vi "Action Worker Mode Example.vi"() -> ()   [LabVIEW 2017]
uses:
  user.lib/_NEVSTOP/Communicable State Machine(CSM)/_Support/Typedef/_CSM_Response Source Message.ctl
  user.lib/_NEVSTOP/Communicable State Machine(CSM)/_Support/Typedef/_CSM_MODE.ctl
  user.lib/_NEVSTOP/Communicable State Machine(CSM)/AdvanceAPI/CSM - Break Down Multiple States String.vi
  user.lib/_NEVSTOP/Communicable State Machine(CSM)/AdvanceAPI/CSM - Compact Multiple States.vi
  user.lib/_NEVSTOP/Communicable State Machine(CSM)/AdvanceAPI/CSM - Make String Arguments Safe.vi
  user.lib/_NEVSTOP/Communicable State Machine(CSM)/AdvanceAPI/CSM - Keywords.vi
  user.lib/_NEVSTOP/Communicable State Machine(CSM)/_Support/CSMQ/_CSMOFGV.vi
  user.lib/_NEVSTOP/Communicable State Machine(CSM)/_Support/FGV-BroadcastRegistry/global-CSMQ FGV Change Flag.vi
  user.lib/_NEVSTOP/Communicable State Machine(CSM)/Communicable State Machine.lvlib
panel:
  in  "All?":bool
  out "Array":T2(array[cluster])
  out ">> Response Source Message >>":T3
  in  "DoSth: Error -> Worker":bool
  in  "DoSth: Error -@ Worker":bool
  in  "Macro: Exit -> Worker":bool
  in  "Macro: Exit -@ Worker":bool
  in  "DoSth: DoA -@ Worker":bool
  out "State History":string
  in  "DoSth: DoA -> Worker":bool
  # "Overview:\n\nThis demonstrates the worker mode in the CSM framework. Worker mode involves starting multiple clonable instances of CSM, which work together as sub-modules. Normally, if we use the same name for cloneable modules, a critical error will occur in the subsequently started instance. To distinguish it from normal cases, CSM uses a # postfix in module names. Suppose the workers are named with \"worker#\". If you try to send a message to \"worker\", the first idle instance will respond to the message. The term \"FIRST IDLE\" refers to using a fairy queue for waiting instances. From outside, you won't even know that 4 worker instances are running. All concepts of CSM remain unchanged in worker mode, including sync/async/status messages.\n\nIn this example, 4 worker instances of “worker” are running in the background. Please refer to the history log to identify which instance processed your message."
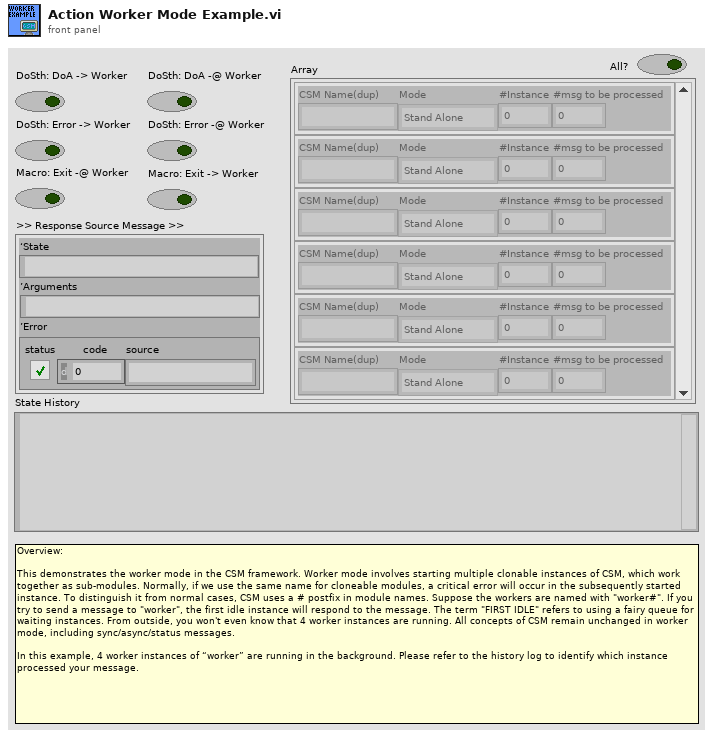
[diagram p1: front panel]
types:
  T1 = typedef "Communicable State Machine.lvlib/_CSM_MODE.ctl" = enum16{"Not Exist", "Stand Alone", "CSM", "Worker Agent", "Worker", "Chain", "Chain Node"}
  T2 = cluster{"CSM Name(dup)":string, "Mode":T1, "#Instance":i32, "#msg to be processed":i32}[]
  T3 = typedef "Communicable State Machine.lvlib/_CSM_Response Source Message.ctl" = cluster{"‘State":string, "’Arguments":string, "’Error":errorcluster}
  T4 = enum32{"Invalid", "Standard", "Closed", "Hidden", "Minimized", "Maximized"}
  T5 = enum32{"invalid app kind", "Development System", "Run Time System", "Student Edition", "Embedded LabVIEW", "Evaluation", "Custom"}
  T6 = cluster{"Current VI Reference":refnum<vi>, "Close Panel on Exit?":bool}
  T7 = cluster{"Core":cluster{"Current VI Reference":refnum<vi>, "Close Panel on Exit?":bool}, "Your Boolean data":bool, "Your string data":string}
  T8 = cluster{"CSM Name(dup)":string, "Mode":T1, "#Instance":i32, "#msg to be processed":i32}
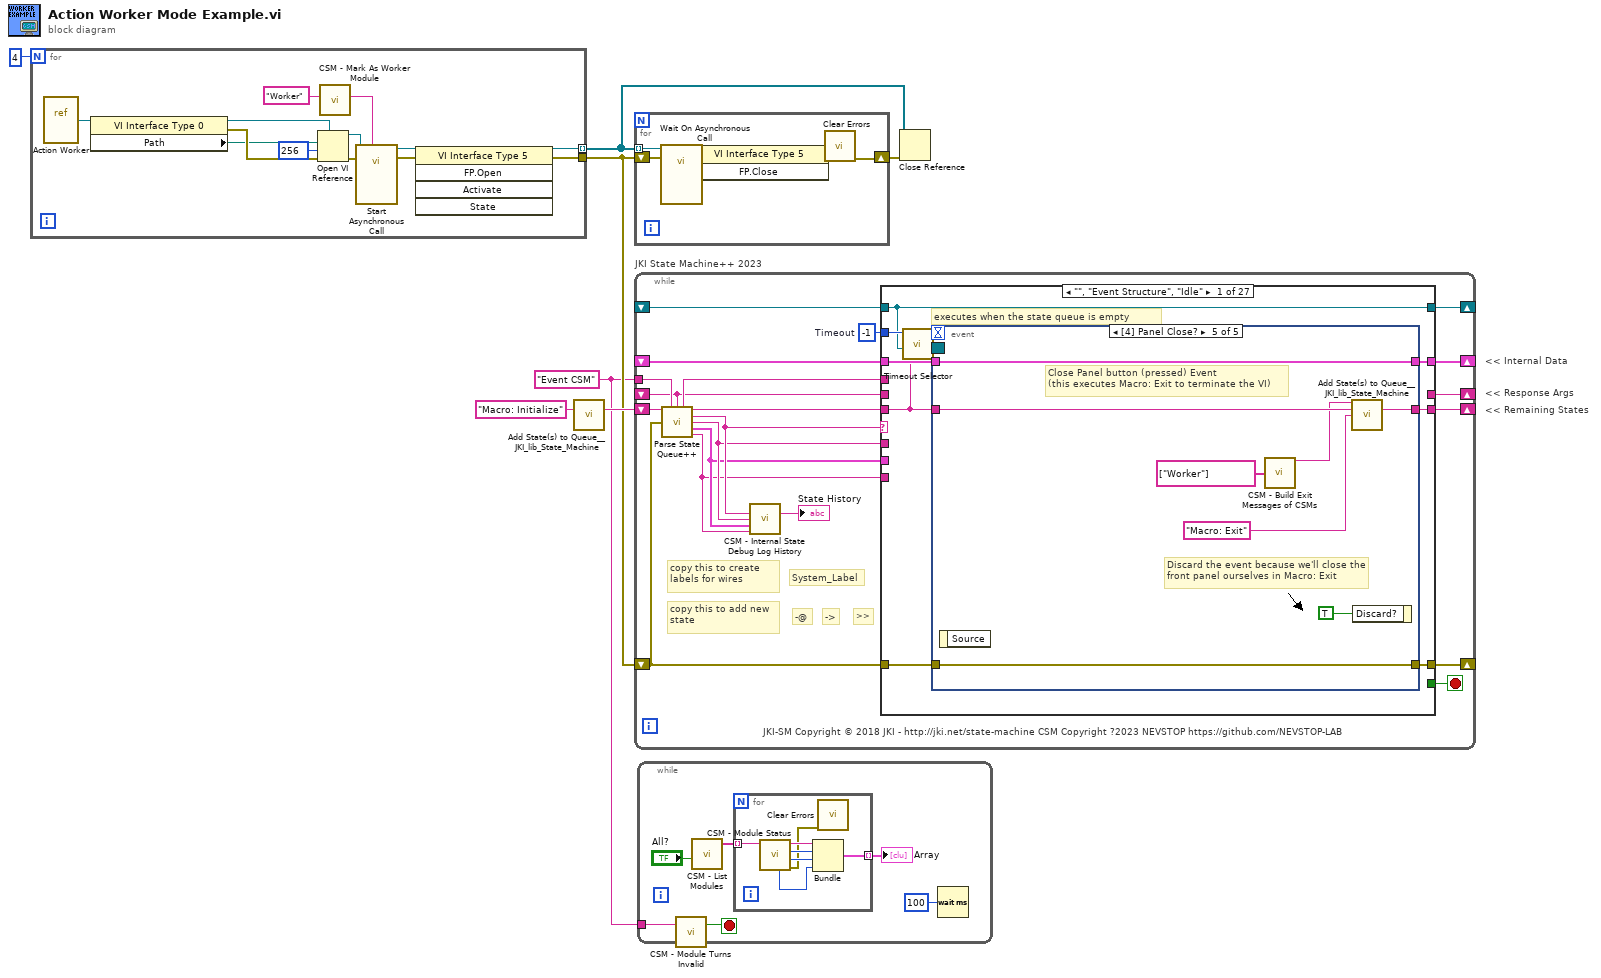
[diagram p0: block diagram]
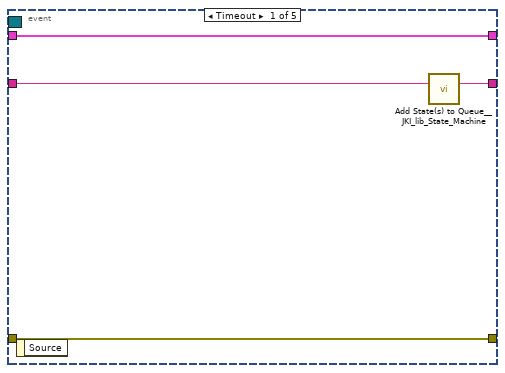
[diagram p2: hidden frame]
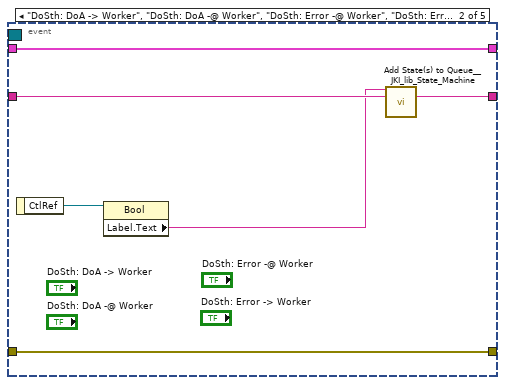
[diagram p3: hidden frame]
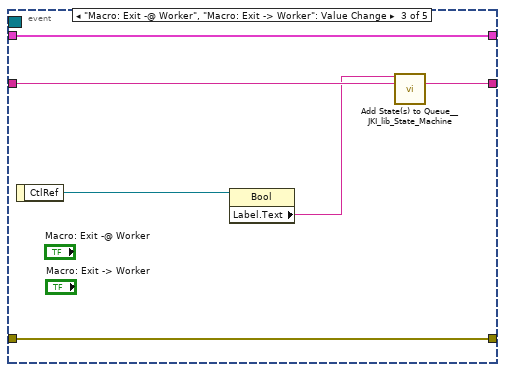
[diagram p4: hidden frame]
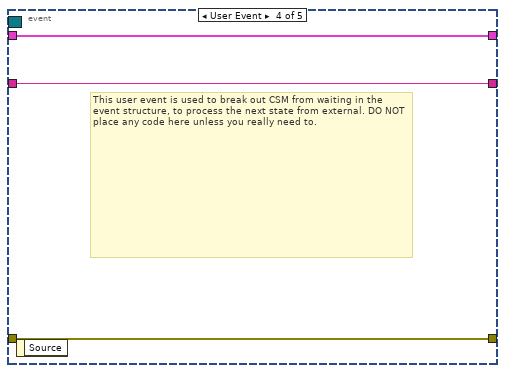
[diagram p5: hidden frame]
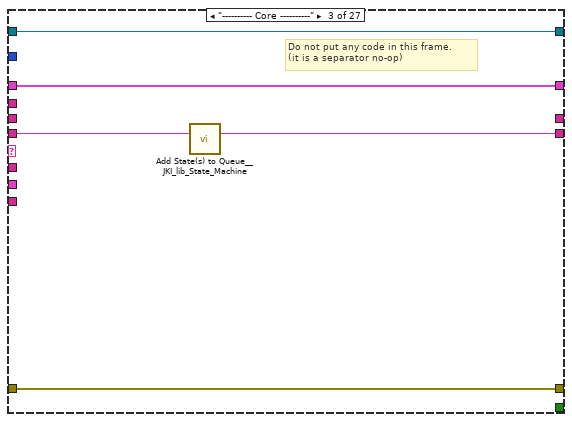
[diagram p7: hidden frame]
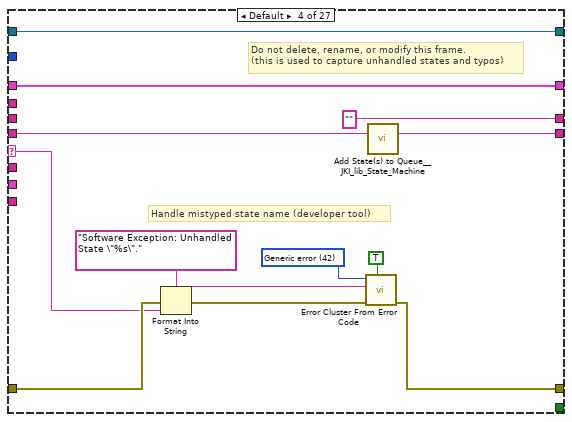
[diagram p8: hidden frame]
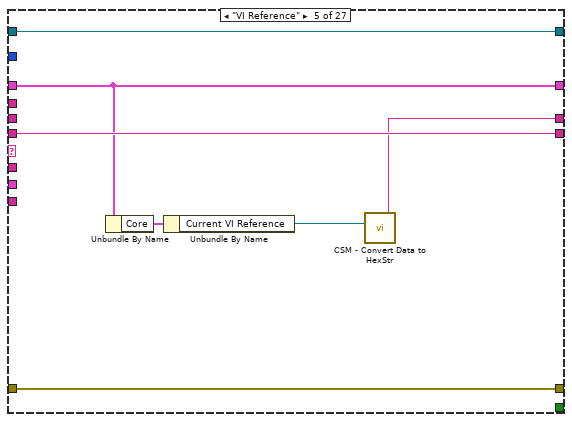
[diagram p9: hidden frame]
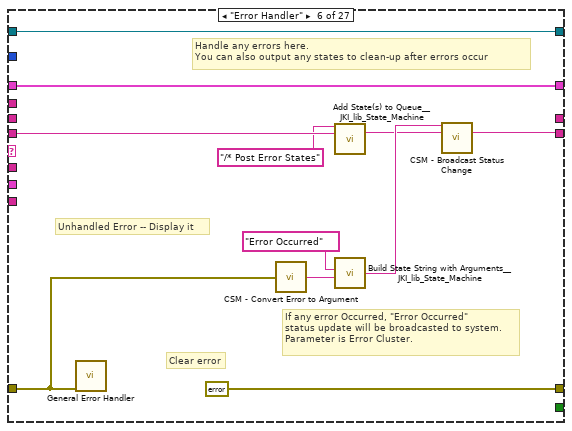
[diagram p10: hidden frame]
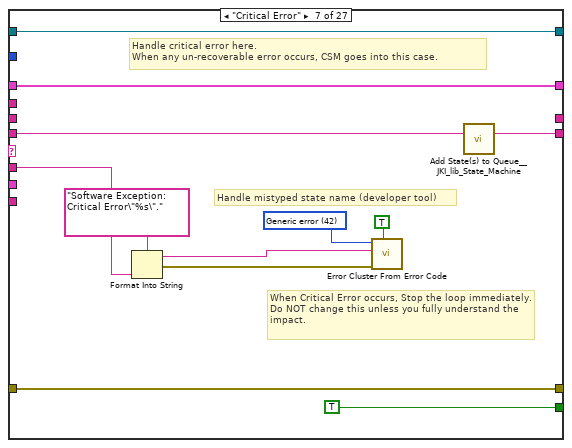
[diagram p11: hidden frame]
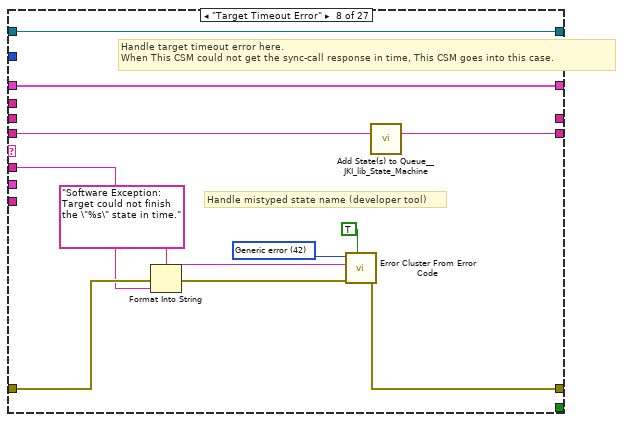
[diagram p12: hidden frame]
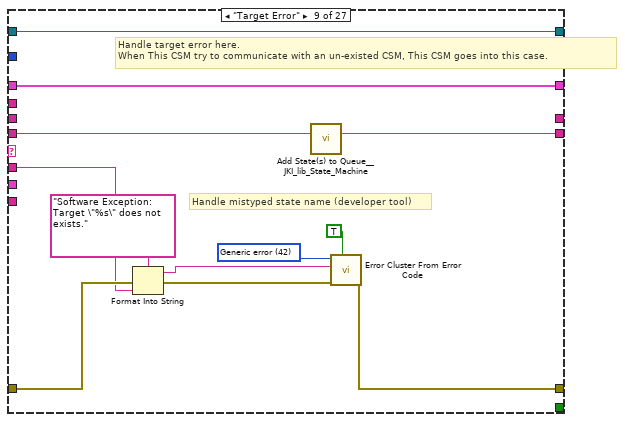
[diagram p13: hidden frame]
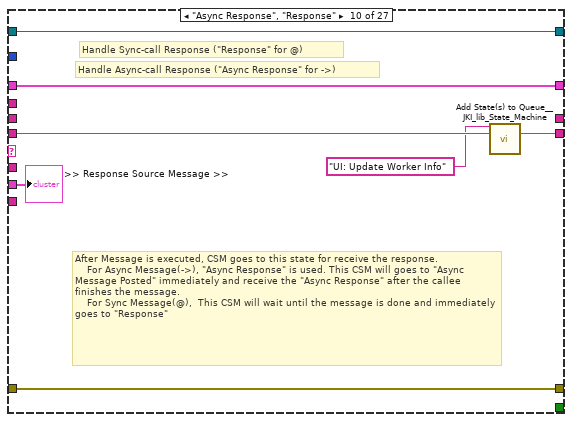
[diagram p14: hidden frame]
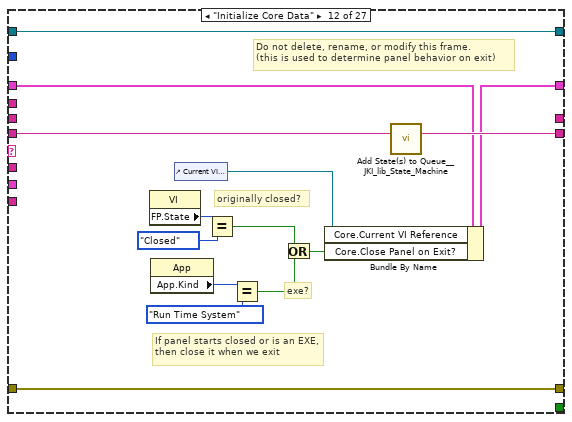
[diagram p16: hidden frame]
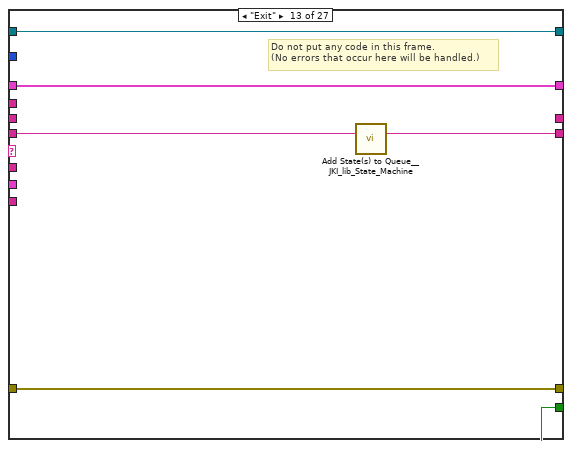
[diagram p17: hidden frame]
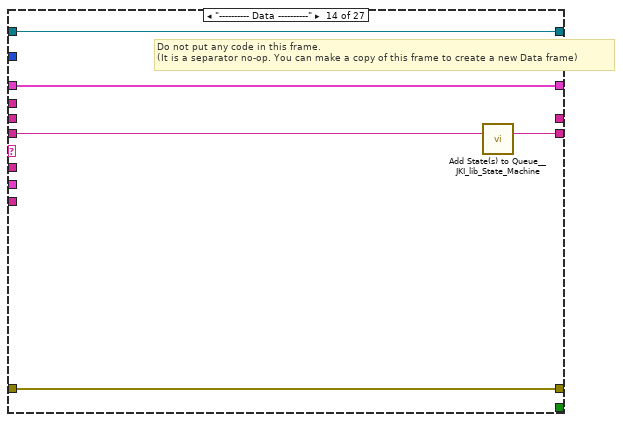
[diagram p18: hidden frame]
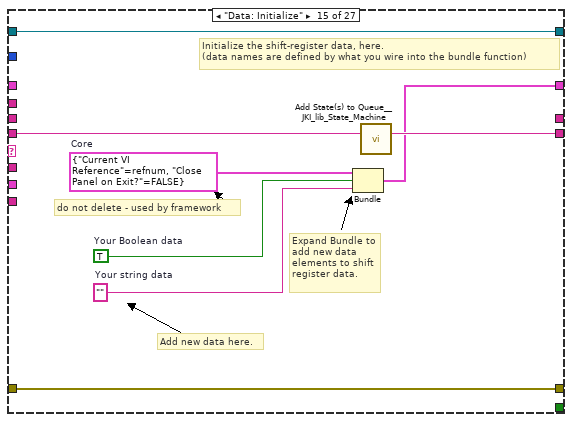
[diagram p19: hidden frame]
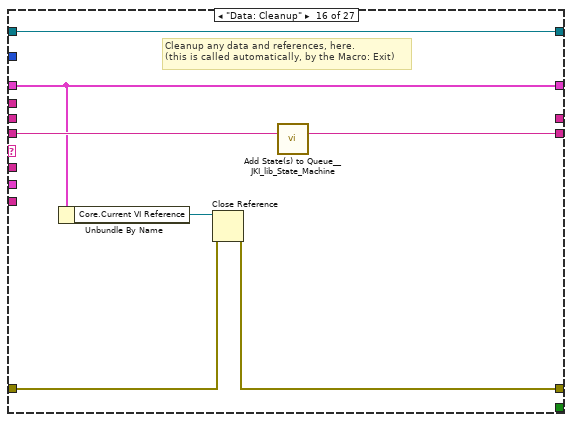
[diagram p20: hidden frame]
diagram:
  w1 = "Event CSM" ("Name(\"\" to use uuid)")
  # "<< Internal Data"
  # "<< Response Args"
  # "<< Remaining States"
  n1 = for {
    N: 4 -> [_]
    tunnel: [w11] -> w2
    tunnel: [w12] -> w3 mode=indexing
    n2 = vi-ref "Action Worker.vi"() -> (w15:refnum<vi>)
    n3 = property class="VI Interface Type 0"(reference=w15) -> (reference out=w19:refnum<vi>, error out=w17:errorcluster, "Path"=w16:path)  [unwired: 1 in]
    n4 = Open VI Reference(type specifier VI Refnum (for type only)=w19, vi path=w16, options=256, error in (no error)=w17) -> (vi reference=w18:refnum<vi>, error out=w14:errorcluster)  [unwired: 2 in]
    n5 = call "CSM - Mark As Worker Module.vi"("CSM Name"="Worker" ("Name(\"\" to use uuid)")) -> ("CSM Name(marked as worker)"=w8:string)  [unwired: 9 in]
    n6 = call-by-ref "Start Asynchronous Call"(reference=w18, error in=w14, "Name(\"\" to use uuid)"=w8) -> (reference out=w13:refnum<vi>, error out=w10:errorcluster)  [unwired: 11 in]
    n7 = invoke class="VI Interface Type 5" method="FP.Open"(reference=w13, error in=w10) -> (reference out=w12:refnum<vi>, error out=w11:errorcluster)  [unwired: 3 in, 3 out]
  }
  n8 = call <vilib>:"Add State(s) to Queue__JKI_lib_State_Machine.vi"("State(s) in (\"\")"="Macro: Initialize") -> ("States Out"=w7:string)  [unwired: 14 in]
  n9 = for {
    shift-right: [w21] -> w5
    shift-left: w2 -> [w26]
    tunnel: w3 -> [w25] mode=indexing
    n10 = call-by-ref "Wait On Asynchronous Call"(reference=w25, error in=w26) -> (reference out=w24:refnum<vi>, error out=w22:errorcluster)  [unwired: 12 in]
    n11 = invoke class="VI Interface Type 5" method="FP.Close"(reference=w24, error in=w22) -> (error out=w23:errorcluster)  [unwired: 1 in, 2 out]
    n12 = call <vilib>:"Clear Errors.vi"("error in (no error)"=w23) -> ("error out"=w21:errorcluster)  [unwired: 5 in, 1 out]
  }
  n13 = while "JKI State Machine++ 2023" {
    shift-right: [w41] -> _
    shift-left: _ -> [w40]
    shift-right: [w44] -> _
    shift-left: w2 -> [w38]
    shift-right: [w43] -> _
    shift-left: w7 -> [w45]
    tunnel: w1 -> [w34]
    shift-right: [w37] -> _
    shift-left: _ -> [w28]
    shift-right: [w36] -> _
    shift-left: _ -> [w35]
    stop <- w42 stop-if-true
    w39 = -1  # Timeout
    # "JKI-SM Copyright © 2018 JKI - http://jki.net/state-machine CSM Copyright ?2023 NEVSTOP https://github.com/NEVSTOP-LAB"
    # "copy this to add new state"
    # ">>"
    # "->"
    # "-@"
    # "copy this to create labels for wires"
    # "System_Label"
    n14 = call "Parse State Queue++.vi"("State Queue"=w45, "Name(\"\" to use uuid)"=w34, "Response Arguments"=w28, "Previous Error"=w38) -> ("Name Used"=w29:string, "Remaining States"=w46:string, "Current State"=w33:string, "Arguments"=w32:string, ">> Response Source Message >>"=w31:T3, ">> Source CSM >>"=w30:string)  [unwired: 6 in]
    n15 = call "CSM - Internal State Debug Log History.vi"("State"=w33, "Arguments (\"\")"=w32, ">> Response Source Message >>"=w31, "Source (\"\")"=w30) -> ("Debug Log"=→"State History":string)  [unwired: 11 in]
    n16 = case shown="\"\", \"Event Structure\", \"Idle\"" w33 {
      selector: w33 -> [_ _ _ w94 _ _ _ _ _ _ _ _ _ _ _ _ _ _ _ _ _ _ _ _ _ _ _]
      tunnel: w46 -> [w47 w85 w91 w98 w110 w122 w132 w140 w152 w162 w168 w183 w189 w194 w202 w209 w214 w220 w224 w230 w235 w242 w258 w326 w332 w338 w349]
      tunnel: w32 -> [_ _ _ _ _ _ w125 w136 w148 _ _ _ _ _ _ _ _ _ _ _ _ w237 w252 _ _ _ _]
      tunnel: w40 -> [w54 w84 w88 w96 w109 w120 w133 w138 w150 w164 w167 w176 w187 w191 _ w204 w211 w219 w223 w227 w233 w240 w254 w325 w329 w335 w346]
      tunnel: [w53 w86 w89 w100 w111 errorcluster {"status"=FALSE, "code"=0, "source"=""} ("error out") w134 w142 w154 w165 w169 w180 w186 w192 w199 w205 w212 w215 w222 w228 w232 w238 w255 w327 w330 w336 w347] -> w44
      tunnel: w38 -> [w52 w86 w89 w99 w111 w112 w134 w141 w153 w165 w169 w180 w186 w192 w199 w206 w212 _ w225 w228 w232 w239 w256 w327 w330 w336 w347]
      tunnel: [w55 w85 w90 w97 w110 w113 w131 w139 w151 w161 w168 w182 w188 w193 w201 w208 w213 w220 w224 w229 w234 w241 w257 w326 w331 w337 w348] -> w43
      tunnel: [_ _ _ _ _ _ TRUE _ _ _ _ _ TRUE _ _ _ _ _ _ _ _ _ _ _ _ _ _] -> w42
      tunnel: [w51 w84 w88 w96 w109 w120 w133 w138 w150 w164 w167 w181 w187 w191 w200 w204 w211 w219 w223 w227 w233 w240 w254 w325 w329 w335 w346] -> w41
      tunnel: w39 -> [w50 _ _ _ _ _ _ _ _ _ _ _ _ _ _ _ _ _ _ _ _ _ _ _ _ _ _]
      tunnel: w30 -> [_ _ _ _ _ _ _ _ _ _ _ _ _ _ _ _ _ _ _ _ _ _ _ _ _ _ _]
      tunnel: w31 -> [_ _ _ _ _ _ _ _ _ w159 _ _ _ _ _ _ _ _ _ _ _ _ _ _ _ _ _]
      tunnel: [_ _ _ "" w105 _ _ _ _ _ _ _ _ _ _ _ _ _ _ _ _ _ _ _ _ _ _] -> w37
      tunnel: [w49 w83 w87 w92 w108 w118 w123 w135 w147 w163 w166 w170 w184 w190 w195 w203 w210 w218 w221 w226 w231 w236 w251 w324 w328 w333 w339] -> w36
      tunnel: w35 -> [w49 w83 w87 w92 w108 w118 w123 w135 w147 w163 w166 w170 w184 w190 w195 w203 w210 _ w221 w226 w231 w236 w251 w324 w328 w333 w339]
      tunnel: w29 -> [_ _ _ _ _ _ _ _ _ _ _ _ _ _ _ _ _ w217 _ _ _ _ _ _ _ _ _]
      tunnel: w28 -> [_ _ _ _ _ _ _ _ _ _ _ _ _ _ _ _ _ _ _ _ _ _ _ _ _ _ _]
      frame "", "Event Structure", "Idle" {
        # "executes when the state queue is empty"
        n17 = call "Timeout Selector.vi"("Remaining States"=w47, "Timeout Expected"=w50) -> ("Timeout"=w48:i32)  [unwired: 5 in]
        n18 = event shown="[4] Panel Close?" {
          selector: w49 -> [_ _ _ _ _]
          dyn-events: _ -> [_ _ _ _ _]
          timeout: w48 -> [_ _ _ _ _]
          tunnel: w47 -> [w59 w63 w69 w73 w82]
          tunnel: [w58 w62 w68 w73 w81] -> w55
          tunnel: w54 -> [w56 w64 w70 w74 w79]
          tunnel: [w57 w65 w71 w72 w80] -> w53
          tunnel: w52 -> [w57 w65 w71 w72 w80]
          tunnel: [w56 w64 w70 w74 w79] -> w51
          event Timeout {
            n19 = event-data() -> ()  [unwired: 1 in, 1 out]
            n20 = call <vilib>:"Add State(s) to Queue__JKI_lib_State_Machine.vi"("State(s) in (\"\")"=w59) -> ("States Out"=w58:string)  [unwired: 14 in]
          }
          event "DoSth: DoA -> Worker", "DoSth: DoA -@ Worker", "DoSth: Error -@ Worker", "DoSth: Error -> Worker": Value Change {
            n21 = event-data() -> ("CtlRef"=w61:refnum<vi>)  [unwired: 1 in]
            n22 = property class="Bool"(reference=w61) -> ("Label.Text"=w60:string)  [unwired: 1 in, 2 out]
            n23 = call <vilib>:"Add State(s) to Queue__JKI_lib_State_Machine.vi"("State(s) in Front (\"\")"=w60, "State(s) in (\"\")"=w63) -> ("States Out"=w62:string)  [unwired: 13 in]
          }
          event "Macro: Exit -@ Worker", "Macro: Exit -> Worker": Value Change {
            n24 = event-data() -> ("CtlRef"=w67:refnum<vi>)  [unwired: 1 in]
            n25 = property class="Bool"(reference=w67) -> ("Label.Text"=w66:string)  [unwired: 1 in, 2 out]
            n26 = call <vilib>:"Add State(s) to Queue__JKI_lib_State_Machine.vi"("State(s) in Front (\"\")"=w66, "State(s) in (\"\")"=w69) -> ("States Out"=w68:string)  [unwired: 13 in]
          }
          event User Event {
            # "This user event is used to break out CSM from waiting in the event structure, to process the next state from external. DO NOT place any code here unless you really need to."
            n27 = event-data() -> ()  [unwired: 1 in, 1 out]
          }
          event Panel Close? {
            # "Discard the event because we'll close the front panel ourselves in Macro: Exit"
            # "Close Panel button (pressed) Event\n(this executes Macro: Exit to terminate the VI)"
            n28 = event-data() -> ()  [unwired: 1 in, 1 out]
            n29 = call "CSM - Build Exit Messages of CSMs.vi"("CSMs"=string[] ["Worker"]) -> ("States"=w76:string)  [unwired: 14 in]
            n30 = call <vilib>:"Add State(s) to Queue__JKI_lib_State_Machine.vi"("State(s) in Front (\"\")"=w76, "State(s) in (\"\")"=w82, "State(s) at Back (\"\")"="Macro: Exit") -> ("States Out"=w81:string)  [unwired: 12 in]
            n31 = event-data("Discard?"=TRUE) -> ()  [unwired: 1 in, 1 out]
          }
        }
      }
      frame "CSM Documentation" {
        # "#CSM README FIRST\n\nCSM is a LabVIEW application framework that builds upon JKI State Machine (JKISM). It follows the pattern of JKISM and extends the keywords to describe message communication between CSM modules, including concepts such as Sync-Message, Async-Message, Subscription/Unsubscription of status - essential elements for creating reusable code modules. For more information, please visit the CSM wiki: https://github.com/NEVSTOP-LAB/JKI-State-Machine-Plus-Plus/wiki\n\nFor instructions on JKI State Machine, visit: http://jki.net/state-machine/\nFor information about CSM, visit: https://github.com/NEVSTOP-LAB"
        # "CSM Documentation"
      }
      frame "---------- Core ----------" {
        # "Do not put any code in this frame.\n(it is a separator no-op)"
        n32 = call <vilib>:"Add State(s) to Queue__JKI_lib_State_Machine.vi"("State(s) in (\"\")"=w91) -> ("States Out"=w90:string)  [unwired: 14 in]
      }
      frame Default {
        w103 = 42 items=["No error", "Argument error", "Memory is full", "Out of zone", "End of file", "File already open", "Generic file I/O error", "File not found", "File permission error", "Disk is full", "Duplicate path", "Too many files open", "System feature not enabled", "Resource file not found", "Cannot add resource", "Resource not found", "Image not found", "Image memory error", "Pen does not exist", "Config type invalid", "Config token not found", "Config parse error", "Config memory error", "Bad external code format", "Bad external code offset", "External code not present", "Null window", "Destroy window error", "Null menu", "Print aborted", "Bad print record", "Print driver error", "Windows error during printing", "Memory error during printing", "Print dialog error", "Generic print error", "Invalid device refnum", "Device not found", "Device parameter error", "Device unit error", "Cannot open device", "Device call aborted", "Generic error", "Cancelled by user", "Object ID too low", "Object ID too high", "Object not in heap", "Unknown heap", "Unknown object (invalid DefProc)", "Unknown object (DefProc not in table)", "Message out of range", "Invalid (null) method", "Unknown message", "Manager call not supported", "Bad address", "Network operation in progress", "Network operation timed out", "Connection is busy", "Network attribute not supported", "Network error", "Address in use", "System out of memory", "Connection aborted", "Connection refused", "Not connected", "Already connected", "Connection closed", "Initialization error (interapplication manager)", "Bad occurrence", "Wait on unbound occurrence handler", "Occurrence queue overflow", "Datalog type conflict", "Unused", "Unrecognized type (interapplication manager)", "Memory corrupt", "Failed to make temporary DLL", "Old CIN version", "Drag socket not found", "Failed to load drop-object", "Failed to register OLE object", "Failed to release OLE object", "Format specifier type mismatch", "Unknown format specifier", "Too few format specifiers", "Too many format specifiers", "Scan failed", "Newer CIN version", "Error converting to variant", "Runtime menu error", "Password tampered", "Variant attribute not found", "Incompatible variant data type", "Event data is not available", "Event Store is not present", "Occurrence is not found", "Event Queue is not created", "Event info is not available", "Refnum passed is NULL", "Error retrieving Class GUID", "Error retrieving CoClass GUID", "Error retrieving TypeLib GUID.", "Bad built application magic bytes.", "Specific driver is different from the specific driver associated with the Logical Name.", "There is no session opened to the class driver.", "Max Error", "MAX - Error with config objects", "MAX - Error loading configuration", "MAX - Group not supported"]
        # "Do not delete, rename, or modify this frame.\n(this is used to capture unhandled states and typos)"
        # "Handle mistyped state name (developer tool)"
        n33 = Format Into String(format string="Software Exception: Unhandled State \"%s\"." ("message"), error in=w99, w94) -> (resulting string=w102:string, error out=w101:errorcluster)  [unwired: 1 in]
        n34 = call <vilib>:"Error Cluster From Error Code.vi"("show call chain? (False)"=TRUE, "error in (no error)"=w101, "error message (\"\")"=w102, "error code (0)"=w103) -> ("error out"=w100:errorcluster)  [unwired: 5 in]
        n35 = call <vilib>:"Add State(s) to Queue__JKI_lib_State_Machine.vi"("State(s) in (\"\")"=w98) -> ("States Out"=w97:string)  [unwired: 14 in]
      }
      frame "VI Reference" {
        n36 = Unbundle By Name(w109) -> ("Core"=w107:T6)
        n37 = Unbundle By Name(w107) -> ("Current VI Reference"=w106:refnum<vi>)
        n38 = call "CSM - Convert Data to HexStr.vi"("Variant"=w106) -> ("HEX String (0-9,A-F)"=w105:string)  [unwired: 8 in]
      }
      frame "Error Handler" {
        # "If any error Occurred, \"Error Occurred\" \nstatus update will be broadcasted to system.\nParameter is Error Cluster."
        # "Unhandled Error -- Display it"
        # "Handle any errors here.\nYou can also output any states to clean-up after errors occur"
        # "Clear error"
        n39 = call <vilib>:"General Error Handler.vi"("error in (no error)"=w112) -> ()  [unwired: 10 in, 5 out]
        n40 = call "CSM - Convert Error to Argument.vi"("error"=w112) -> ("Argument"=w116:string)  [unwired: 4 in]
        n41 = call <vilib>:"Add State(s) to Queue__JKI_lib_State_Machine.vi"("State(s) in Front (\"\")"="/* Post Error States", "State(s) in (\"\")"=w122) -> ("States Out"=w114:string)  [unwired: 13 in]
        n42 = call <vilib>:"Build State String with Arguments__JKI_lib_State_Machine.vi"("Arguments (\"\")"=w116, "State"="Error Occurred" ("Status with Arguments")) -> ("State with Arguments"=w115:string)  [unwired: 4 in]
        n43 = call "CSM - Broadcast Status Change.vi"("Status with Arguments"=w115, "State Queue"=w114) -> ("Remaining States"=w113:string)  [unwired: 13 in]
      }
      frame "Critical Error" {
        w129 = 42 items=["No error", "Argument error", "Memory is full", "Out of zone", "End of file", "File already open", "Generic file I/O error", "File not found", "File permission error", "Disk is full", "Duplicate path", "Too many files open", "System feature not enabled", "Resource file not found", "Cannot add resource", "Resource not found", "Image not found", "Image memory error", "Pen does not exist", "Config type invalid", "Config token not found", "Config parse error", "Config memory error", "Bad external code format", "Bad external code offset", "External code not present", "Null window", "Destroy window error", "Null menu", "Print aborted", "Bad print record", "Print driver error", "Windows error during printing", "Memory error during printing", "Print dialog error", "Generic print error", "Invalid device refnum", "Device not found", "Device parameter error", "Device unit error", "Cannot open device", "Device call aborted", "Generic error", "Cancelled by user", "Object ID too low", "Object ID too high", "Object not in heap", "Unknown heap", "Unknown object (invalid DefProc)", "Unknown object (DefProc not in table)", "Message out of range", "Invalid (null) method", "Unknown message", "Manager call not supported", "Bad address", "Network operation in progress", "Network operation timed out", "Connection is busy", "Network attribute not supported", "Network error", "Address in use", "System out of memory", "Connection aborted", "Connection refused", "Not connected", "Already connected", "Connection closed", "Initialization error (interapplication manager)", "Bad occurrence", "Wait on unbound occurrence handler", "Occurrence queue overflow", "Datalog type conflict", "Unused", "Unrecognized type (interapplication manager)", "Memory corrupt", "Failed to make temporary DLL", "Old CIN version", "Drag socket not found", "Failed to load drop-object", "Failed to register OLE object", "Failed to release OLE object", "Format specifier type mismatch", "Unknown format specifier", "Too few format specifiers", "Too many format specifiers", "Scan failed", "Newer CIN version", "Error converting to variant", "Runtime menu error", "Password tampered", "Variant attribute not found", "Incompatible variant data type", "Event data is not available", "Event Store is not present", "Occurrence is not found", "Event Queue is not created", "Event info is not available", "Refnum passed is NULL", "Error retrieving Class GUID", "Error retrieving CoClass GUID", "Error retrieving TypeLib GUID.", "Bad built application magic bytes.", "Specific driver is different from the specific driver associated with the Logical Name.", "There is no session opened to the class driver.", "Max Error", "MAX - Error with config objects", "MAX - Error loading configuration", "MAX - Group not supported"]
        # "Handle critical error here.\nWhen any un-recoverable error occurs, CSM goes into this case."
        # "When Critical Error occurs, Stop the loop immediately. Do NOT change this unless you fully understand the impact."
        # "Handle mistyped state name (developer tool)"
        n44 = Format Into String(format string="Software Exception: Critical Error\"%s\"." ("message"), w125) -> (resulting string=w128:string, error out=w127:errorcluster)  [unwired: 2 in]
        n45 = call <vilib>:"Error Cluster From Error Code.vi"("show call chain? (False)"=TRUE, "error in (no error)"=w127, "error message (\"\")"=w128, "error code (0)"=w129) -> ()  [unwired: 5 in, 1 out]
        n46 = call <vilib>:"Add State(s) to Queue__JKI_lib_State_Machine.vi"("State(s) in (\"\")"=w132) -> ("States Out"=w131:string)  [unwired: 14 in]
      }
      frame "Target Timeout Error" {
        w145 = 42 items=["No error", "Argument error", "Memory is full", "Out of zone", "End of file", "File already open", "Generic file I/O error", "File not found", "File permission error", "Disk is full", "Duplicate path", "Too many files open", "System feature not enabled", "Resource file not found", "Cannot add resource", "Resource not found", "Image not found", "Image memory error", "Pen does not exist", "Config type invalid", "Config token not found", "Config parse error", "Config memory error", "Bad external code format", "Bad external code offset", "External code not present", "Null window", "Destroy window error", "Null menu", "Print aborted", "Bad print record", "Print driver error", "Windows error during printing", "Memory error during printing", "Print dialog error", "Generic print error", "Invalid device refnum", "Device not found", "Device parameter error", "Device unit error", "Cannot open device", "Device call aborted", "Generic error", "Cancelled by user", "Object ID too low", "Object ID too high", "Object not in heap", "Unknown heap", "Unknown object (invalid DefProc)", "Unknown object (DefProc not in table)", "Message out of range", "Invalid (null) method", "Unknown message", "Manager call not supported", "Bad address", "Network operation in progress", "Network operation timed out", "Connection is busy", "Network attribute not supported", "Network error", "Address in use", "System out of memory", "Connection aborted", "Connection refused", "Not connected", "Already connected", "Connection closed", "Initialization error (interapplication manager)", "Bad occurrence", "Wait on unbound occurrence handler", "Occurrence queue overflow", "Datalog type conflict", "Unused", "Unrecognized type (interapplication manager)", "Memory corrupt", "Failed to make temporary DLL", "Old CIN version", "Drag socket not found", "Failed to load drop-object", "Failed to register OLE object", "Failed to release OLE object", "Format specifier type mismatch", "Unknown format specifier", "Too few format specifiers", "Too many format specifiers", "Scan failed", "Newer CIN version", "Error converting to variant", "Runtime menu error", "Password tampered", "Variant attribute not found", "Incompatible variant data type", "Event data is not available", "Event Store is not present", "Occurrence is not found", "Event Queue is not created", "Event info is not available", "Refnum passed is NULL", "Error retrieving Class GUID", "Error retrieving CoClass GUID", "Error retrieving TypeLib GUID.", "Bad built application magic bytes.", "Specific driver is different from the specific driver associated with the Logical Name.", "There is no session opened to the class driver.", "Max Error", "MAX - Error with config objects", "MAX - Error loading configuration", "MAX - Group not supported"]
        # "Handle target timeout error here.\nWhen This CSM could not get the sync-call response in time, This CSM goes into this case."
        # "Handle mistyped state name (developer tool)"
        n47 = Format Into String(format string="Software Exception: Target could not finish the \"%s\" state in time." ("message"), error in=w141, w136) -> (resulting string=w144:string, error out=w143:errorcluster)  [unwired: 1 in]
        n48 = call <vilib>:"Error Cluster From Error Code.vi"("show call chain? (False)"=TRUE, "error in (no error)"=w143, "error message (\"\")"=w144, "error code (0)"=w145) -> ("error out"=w142:errorcluster)  [unwired: 5 in]
        n49 = call <vilib>:"Add State(s) to Queue__JKI_lib_State_Machine.vi"("State(s) in (\"\")"=w140) -> ("States Out"=w139:string)  [unwired: 14 in]
      }
      frame "Target Error" {
        w157 = 42 items=["No error", "Argument error", "Memory is full", "Out of zone", "End of file", "File already open", "Generic file I/O error", "File not found", "File permission error", "Disk is full", "Duplicate path", "Too many files open", "System feature not enabled", "Resource file not found", "Cannot add resource", "Resource not found", "Image not found", "Image memory error", "Pen does not exist", "Config type invalid", "Config token not found", "Config parse error", "Config memory error", "Bad external code format", "Bad external code offset", "External code not present", "Null window", "Destroy window error", "Null menu", "Print aborted", "Bad print record", "Print driver error", "Windows error during printing", "Memory error during printing", "Print dialog error", "Generic print error", "Invalid device refnum", "Device not found", "Device parameter error", "Device unit error", "Cannot open device", "Device call aborted", "Generic error", "Cancelled by user", "Object ID too low", "Object ID too high", "Object not in heap", "Unknown heap", "Unknown object (invalid DefProc)", "Unknown object (DefProc not in table)", "Message out of range", "Invalid (null) method", "Unknown message", "Manager call not supported", "Bad address", "Network operation in progress", "Network operation timed out", "Connection is busy", "Network attribute not supported", "Network error", "Address in use", "System out of memory", "Connection aborted", "Connection refused", "Not connected", "Already connected", "Connection closed", "Initialization error (interapplication manager)", "Bad occurrence", "Wait on unbound occurrence handler", "Occurrence queue overflow", "Datalog type conflict", "Unused", "Unrecognized type (interapplication manager)", "Memory corrupt", "Failed to make temporary DLL", "Old CIN version", "Drag socket not found", "Failed to load drop-object", "Failed to register OLE object", "Failed to release OLE object", "Format specifier type mismatch", "Unknown format specifier", "Too few format specifiers", "Too many format specifiers", "Scan failed", "Newer CIN version", "Error converting to variant", "Runtime menu error", "Password tampered", "Variant attribute not found", "Incompatible variant data type", "Event data is not available", "Event Store is not present", "Occurrence is not found", "Event Queue is not created", "Event info is not available", "Refnum passed is NULL", "Error retrieving Class GUID", "Error retrieving CoClass GUID", "Error retrieving TypeLib GUID.", "Bad built application magic bytes.", "Specific driver is different from the specific driver associated with the Logical Name.", "There is no session opened to the class driver.", "Max Error", "MAX - Error with config objects", "MAX - Error loading configuration", "MAX - Group not supported"]
        # "Handle target error here.\nWhen This CSM try to communicate with an un-existed CSM, This CSM goes into this case."
        # "Handle mistyped state name (developer tool)"
        n50 = Format Into String(format string="Software Exception: Target \"%s\" does not exists." ("message"), error in=w153, w148) -> (resulting string=w156:string, error out=w155:errorcluster)  [unwired: 1 in]
        n51 = call <vilib>:"Add State(s) to Queue__JKI_lib_State_Machine.vi"("State(s) in (\"\")"=w152) -> ("States Out"=w151:string)  [unwired: 14 in]
        n52 = call <vilib>:"Error Cluster From Error Code.vi"("show call chain? (False)"=TRUE, "error in (no error)"=w155, "error message (\"\")"=w156, "error code (0)"=w157) -> ("error out"=w154:errorcluster)  [unwired: 5 in]
      }
      frame "Async Response", "Response" {
        # "Handle Async-call Response (\"Async Response\" for ->)"
        # "Handle Sync-call Response (\"Response\" for @)"
        # "After Message is executed, CSM goes to this state for receive the response. \n    For Async Message(->), \"Async Response\" is used. This CSM will goes to \"Async Message Posted\" immediately and receive the \"Async Response\" after the callee finishes the message.\n    For Sync Message(@),  This CSM will wait until the message is done and immediately goes to \"Response\""
        n53 = call <vilib>:"Add State(s) to Queue__JKI_lib_State_Machine.vi"("State(s) in Front (\"\")"="UI: Update Worker Info" ("State(s) at Back (\"\")"), "State(s) in (\"\")"=w162) -> ("States Out"=w161:string)  [unwired: 13 in]
        ">> Response Source Message >>" <- w159
      }
      frame "Async Message Posted" {
        # "Handle post action for async message (->)."
        # "After Async Message is posted (->), CSM goes to this state for post-action. You can use Argument - State to tell which Async Message is called."
      }
      frame "Initialize Core Data" {
        # "Do not delete, rename, or modify this frame.\n(this is used to determine panel behavior on exit)"
        # "originally closed?"
        # "exe?"
        # "If panel starts closed or is an EXE, then close it when we exit"
        n54 = property class="VI"() -> ("FP.State"=w173:T4)  [unwired: 2 in, 2 out]
        n55 = property class="App"() -> ("App.Kind"=w179:T5)  [unwired: 2 in, 2 out]
        n56 = control-ref of="Current VI Reference"() -> (w174:refnum<vi>)
        n57 = Equal?(x=w173, y=T4."Closed" ("Front Panel Window:State")) -> (x = y?=w171:bool)
        n58 = Equal?(x=w179, y=T5."Run Time System" ("Application:Kind")) -> (x = y?=w177:bool)
        n59 = Or(x=w171, y=w177) -> (x .or. y?=w175:bool)
        n60 = Bundle By Name(cluster=w176, "Core.Current VI Reference"=w174, "Core.Close Panel on Exit?"=w175) -> (w181:T7)
        n61 = call <vilib>:"Add State(s) to Queue__JKI_lib_State_Machine.vi"("State(s) in (\"\")"=w183) -> ("States Out"=w182:string)  [unwired: 14 in]
      }
      frame "Exit" {
        # "Do not put any code in this frame.\n(No errors that occur here will be handled.)"
        n62 = call <vilib>:"Add State(s) to Queue__JKI_lib_State_Machine.vi"("State(s) in (\"\")"=w189) -> ("States Out"=w188:string)  [unwired: 14 in]
      }
      frame "---------- Data ----------" {
        # "Do not put any code in this frame.\n(It is a separator no-op. You can make a copy of this frame to create a new Data frame)"
        n63 = call <vilib>:"Add State(s) to Queue__JKI_lib_State_Machine.vi"("State(s) in (\"\")"=w194) -> ("States Out"=w193:string)  [unwired: 14 in]
      }
      frame "Data: Initialize" {
        w196 = T6 {"Current VI Reference"=refnum, "Close Panel on Exit?"=FALSE}  # Core
        w198 = TRUE  # Your Boolean data
        w197 = ""  # Your string data
        # "do not delete - used by framework"
        # "Expand Bundle to add new data elements to shift register data."
        # "Add new data here."
        # "Initialize the shift-register data, here.\n(data names are defined by what you wire into the bundle function)"
        n64 = Bundle("Core"=w196, "Your Boolean data"=w198, "Your string data"=w197) -> (w200:T7)  [unwired: 1 in]
        n65 = call <vilib>:"Add State(s) to Queue__JKI_lib_State_Machine.vi"("State(s) in (\"\")"=w202) -> ("States Out"=w201:string)  [unwired: 14 in]
      }
      frame "Data: Cleanup" {
        # "Cleanup any data and references, here.\n(this is called automatically, by the Macro: Exit)"
        n66 = Unbundle By Name(w204) -> ("Core.Current VI Reference"=w207:refnum<vi>)
        n67 = Close Reference(reference=w207, error in (no error)=w206) -> (error out=w205:errorcluster)
        n68 = call <vilib>:"Add State(s) to Queue__JKI_lib_State_Machine.vi"("State(s) in (\"\")"=w209) -> ("States Out"=w208:string)  [unwired: 14 in]
      }
      frame "---------- Events ----------" {
        # "Do not put any code in this frame.\n(It is a separator no-op. You can make a copy of this frame to create a new UI frame)"
        n69 = call <vilib>:"Add State(s) to Queue__JKI_lib_State_Machine.vi"("State(s) in (\"\")"=w214) -> ("States Out"=w213:string)  [unwired: 14 in]
      }
      frame "Events: Register" {
        # "Register message event to break Waiting in Event structure."
        n70 = call "CSM - Get New State Notifier Event.vi"("Name(\"\" to use uuid) in"=w217) -> ("Error out"=w215:errorcluster, "New State Notifier Event"=w216:refnum<user-event>)  [unwired: 9 in]
        n71 = register-events(w216) -> (reference out=w218:refnum<event-registration>)  [unwired: 2 in, 1 out]
      }
      frame "Events: Unregister" {
        n72 = Unregister For Events(event registration refnum=w221, error in=w225) -> (error out=w222:errorcluster)
      }
      frame "---------- UI ----------" {
        # "Do not put any code in this frame.\n(It is a separator no-op. You can make a copy of this frame to create a new UI frame)"
        n73 = call <vilib>:"Add State(s) to Queue__JKI_lib_State_Machine.vi"("State(s) in (\"\")"=w230) -> ("States Out"=w229:string)  [unwired: 14 in]
      }
      frame "UI: Initialize" {
        # "Initialize the User Interface, here.\n(this is called automatically, by the Macro: Init)"
        n74 = call <vilib>:"Add State(s) to Queue__JKI_lib_State_Machine.vi"("State(s) in (\"\")"=w235) -> ("States Out"=w234:string)  [unwired: 14 in]
      }
      frame "UI: Cursor Set" {
        # "Argument"
        # "Set and Unset Cursor Busy.\n(Usage: \"UI: Cursor Set >> Busy|Idle\")"
        n75 = disable-structure shown="Default" {
          disable-tunnel: w239 -> [w245 w250]
          disable-tunnel: [w244 w250] -> w238
          disable-tunnel: w237 -> [w243 _]
          frame condition #0 (active) {
            n76 = case shown="\"Idle\", Default" w243 {
              tunnel: w245 -> [w247 w249]
              tunnel: [w246 w248] -> w244
              frame "Idle", Default {
                n77 = call <vilib>:"Unset Busy.vi"("error in (no error)"=w247) -> ("error out"=w246:errorcluster)  [unwired: 10 in]
              }
              frame "Busy" {
                n78 = call <vilib>:"Set Busy.vi"("error in (no error)"=w249) -> ("error out"=w248:errorcluster)  [unwired: 9 in, 1 out]
              }
            }
          }
          frame condition #1 {
          }
        }
        n79 = call <vilib>:"Add State(s) to Queue__JKI_lib_State_Machine.vi"("State(s) in (\"\")"=w242) -> ("States Out"=w241:string)  [unwired: 14 in]
      }
      frame "UI: Front Panel State" {
        # "Argument"
        # "Set Front Panel Open or Closed\n(Usage: \"UI: Front Panel State >> Open|Close\")"
        n80 = Unbundle By Name(w254) -> ("Core.Current VI Reference"=w253:refnum<vi>)
        n81 = call <vilib>:"Add State(s) to Queue__JKI_lib_State_Machine.vi"("State(s) in (\"\")"=w258) -> ("States Out"=w257:string)  [unwired: 14 in]
        n82 = case shown="\"Minimize\", \"Minimized\"" w252 {
          tunnel: w256 -> [w264 w279 w290 w303 w316]
          tunnel: [w266 w280 w292 w305 w318] -> w255
          tunnel: w253 -> [w265 w277 w291 w304 w317]
          frame "Open", "Standard", Default {
            w259 = T4."Standard" ("State")
            n83 = property class="VI"(reference=w265, error in=w264) -> (reference out=w262:refnum<vi>, error out=w263:errorcluster, "FP.State"=w261:T4)
            n84 = Not Equal?(x=w261, y=w259) -> (x != y?=w260:bool)
            n85 = case shown="True" w260 {
              tunnel: [w270 w272] -> w266
              tunnel: w263 -> [w269 w272]
              tunnel: w262 -> [w268 _]
              tunnel: w259 -> [w267 _]
              frame True {
                n86 = invoke class="VI" method="FP.Open"(reference=w268, error in=w269, "Activate"=TRUE, "State"=w267) -> (error out=w270:errorcluster)  [unwired: 1 in, 4 out]
              }
              frame False {
              }
            }
          }
          frame "Close", "Closed" {
            n87 = property class="VI"(reference=w277, error in=w279) -> (reference out=w276:refnum<vi>, error out=w278:errorcluster, "FP.State"=w274:T4)
            n88 = Not Equal?(x=w274, y=T4."Closed" ("Front Panel Window:State")) -> (x != y?=w273:bool)
            n89 = case shown="True" w273 {
              tunnel: [w281 w284] -> w280
              tunnel: w278 -> [w281 w283]
              tunnel: w276 -> [_ w282]
              frame False {
              }
              frame True {
                n90 = invoke class="VI" method="FP.Close"(reference=w282, error in=w283) -> (error out=w284:errorcluster)  [unwired: 1 in, 2 out]
              }
            }
          }
          frame "Hidden", "Hide" {
            w285 = T4."Hidden" ("State")
            n91 = property class="VI"(reference=w291, error in=w290) -> (reference out=w288:refnum<vi>, error out=w289:errorcluster, "FP.State"=w287:T4)
            n92 = Not Equal?(x=w287, y=w285) -> (x != y?=w286:bool)
            n93 = case shown="True" w286 {
              tunnel: [w296 w297] -> w292
              tunnel: w289 -> [w295 w297]
              tunnel: w288 -> [w294 _]
              tunnel: w285 -> [w293 _]
              frame True {
                n94 = invoke class="VI" method="FP.Open"(reference=w294, error in=w295, "State"=w293) -> (error out=w296:errorcluster)  [unwired: 2 in, 4 out]
              }
              frame False {
              }
            }
          }
          frame "Minimize", "Minimized" {
            w298 = T4."Minimized" ("State")
            n95 = property class="VI"(reference=w304, error in=w303) -> (reference out=w301:refnum<vi>, error out=w302:errorcluster, "FP.State"=w300:T4)
            n96 = Not Equal?(x=w300, y=w298) -> (x != y?=w299:bool)
            n97 = case shown="True" w299 {
              tunnel: [w309 w310] -> w305
              tunnel: w302 -> [w308 w310]
              tunnel: w301 -> [w307 _]
              tunnel: w298 -> [w306 _]
              frame True {
                n98 = invoke class="VI" method="FP.Open"(reference=w307, error in=w308, "State"=w306) -> (error out=w309:errorcluster)  [unwired: 2 in, 4 out]
              }
              frame False {
              }
            }
          }
          frame "Maximize", "Maximized" {
            w311 = T4."Maximized" ("State")
            n99 = property class="VI"(reference=w317, error in=w316) -> (reference out=w314:refnum<vi>, error out=w315:errorcluster, "FP.State"=w313:T4)
            n100 = Not Equal?(x=w313, y=w311) -> (x != y?=w312:bool)
            n101 = case shown="True" w312 {
              tunnel: [w322 w323] -> w318
              tunnel: w315 -> [w321 w323]
              tunnel: w314 -> [w320 _]
              tunnel: w311 -> [w319 _]
              frame True {
                n102 = invoke class="VI" method="FP.Open"(reference=w320, error in=w321, "State"=w319) -> (error out=w322:errorcluster)  [unwired: 2 in, 4 out]
              }
              frame False {
              }
            }
          }
        }
      }
      frame "UI: Update Worker Info" {
      }
      frame "---------- Macro ----------" {
        # "Do not put any code in this frame.\n(It is a separator no-op. You can make a copy of this frame to create a new Macro frame)"
        n103 = call <vilib>:"Add State(s) to Queue__JKI_lib_State_Machine.vi"("State(s) in (\"\")"=w332) -> ("States Out"=w331:string)  [unwired: 14 in]
      }
      frame "Macro: Initialize" {
        w334 = "Data: Initialize\nInitialize Core Data\nEvents: Register\nUI: Initialize\nUI: Front Panel State >> Open\nUI: Update Worker Info"  # Data: Initialize Initialize Core Data Events: Register UI: Initialize UI: Front Panel State >> Open UI: Update Worker Info
        # "Initialization Macro\n(This is called once, when the VI starts)"
        n104 = call <vilib>:"Add State(s) to Queue__JKI_lib_State_Machine.vi"("State(s) in Front (\"\")"=w334, "State(s) in (\"\")"=w338) -> ("States Out"=w337:string)  [unwired: 13 in]
      }
      frame "Macro: Exit" {
        # "Exit Macro\n(This is called once, when the VI exits)"
        n105 = Unbundle By Name(w346) -> ("Core.Close Panel on Exit?"=w345:bool)
        n106 = Select(t="UI: Front Panel State >> Close", s=w345, f="") -> (s? t:f=w342:string)
        n107 = call <vilib>:"Add State(s) to Queue__JKI_lib_State_Machine.vi"("State(s) in (\"\")"=w342, "State(s) at Back (\"\")"="Data: Cleanup\nEvents: Unregister\nExit") -> ("States Out"=w340:string)  [unwired: 13 in]
        n108 = call <vilib>:"Add State(s) to Queue__JKI_lib_State_Machine.vi"("State(s) in Front (\"\")"=w340, "State(s) in (\"\")"=w349) -> ("States Out"=w348:string)  [unwired: 13 in]
      }
    }
  }
  n109 = while {
    tunnel: w1 -> [w352]
    stop <- w353 stop-if-true
    n110 = call "CSM - Module Turns Invalid.vi"("CSM Name"=w352) -> ("Turn Invalid(Exit)?"=w353:bool)  [unwired: 2 in]
    n111 = call "CSM - List Modules.vi"("All?"="All?") -> ("Module Names"=w354:string[])  [unwired: 9 in, 1 out]
    n112 = for {
      tunnel: w354 -> [w362] mode=indexing
      tunnel: [w357] -> w355 mode=indexing
      n113 = call "CSM - Module Status.vi"("CSM Name"=w362) -> ("Error out"=w356:errorcluster, "#Instance"=w359:i32, "Mode"=w360:T1, "CSM Name(dup)"=w361:string, "#msg to be processed"=w358:i32)  [unwired: 6 in]
      n114 = Bundle("CSM Name(dup)"=w361, "Mode"=w360, "#Instance"=w359, "#msg to be processed"=w358) -> (w357:T8)  [unwired: 1 in]
      n115 = call <vilib>:"Clear Errors.vi"("error in (no error)"=w356) -> ()  [unwired: 5 in, 2 out]
    }
    "Array" <- w355
    n116 = Wait (ms)(milliseconds to wait=u32 100) -> ()  [unwired: 1 out]
  }
  n117 = Close Reference(reference=w3, error in (no error)=w5) -> ()  [unwired: 1 out]
